vi "CB PWM Test.vi"(5 "HMP4040 Channel Settings":T2={"CH1 Voltage"=24.0, "CH1 Current"=1.0, "CH1 Output"=TRUE, "CH2 Voltage"=24.0, "CH2 Current"=1.0, "CH2 Output"=TRUE, "CH3 Voltage"=24.0, "CH3 Current"=1.0, "CH3 Output"=TRUE, "CH4 Voltage"=24.0, "CH4 Current"=1.0, "CH4 Output"=TRUE, "Master Output"=TRUE} {"CH4 Current" format="%.3f"; "CH4 Voltage" format="%.3f"; "CH3 Current" format="%.3f"; "CH3 Voltage" format="%.3f"; "CH2 Current" format="%.3f"; "CH2 Voltage" format="%.3f"; "CH1 Current" format="%.3f"; "CH1 Voltage" format="%.3f"}, 8 "error in (no error)":errorcluster, 9 "Board Selector":T1, 10 "Message IN":string=" ") -> (0 "error out":errorcluster, 1 "Result (bool)":bool, 2 "Message OUT":string, 3 "ControlBoard OUT":refnum<visa-resource-name>)   [LabVIEW 2022 SP3]
uses:
  HMP4000 Communication/HMP4040_ChannelControl.ctl
  Serial Board Com/Board Select.ctl
  <vilib>/DAQmx/read.llb/DAQmx Read (Analog 1D Wfm NChan NSamp).vi
  <vilib>/DAQmx/miscellaneous.llb/DAQmx Fill In Error Info.vi
panel:
  out "Analysis Leg":i32
  out "Waveforms":T3
  out "Active Leg":i32
  out "Result (color)":u32(colorbox)
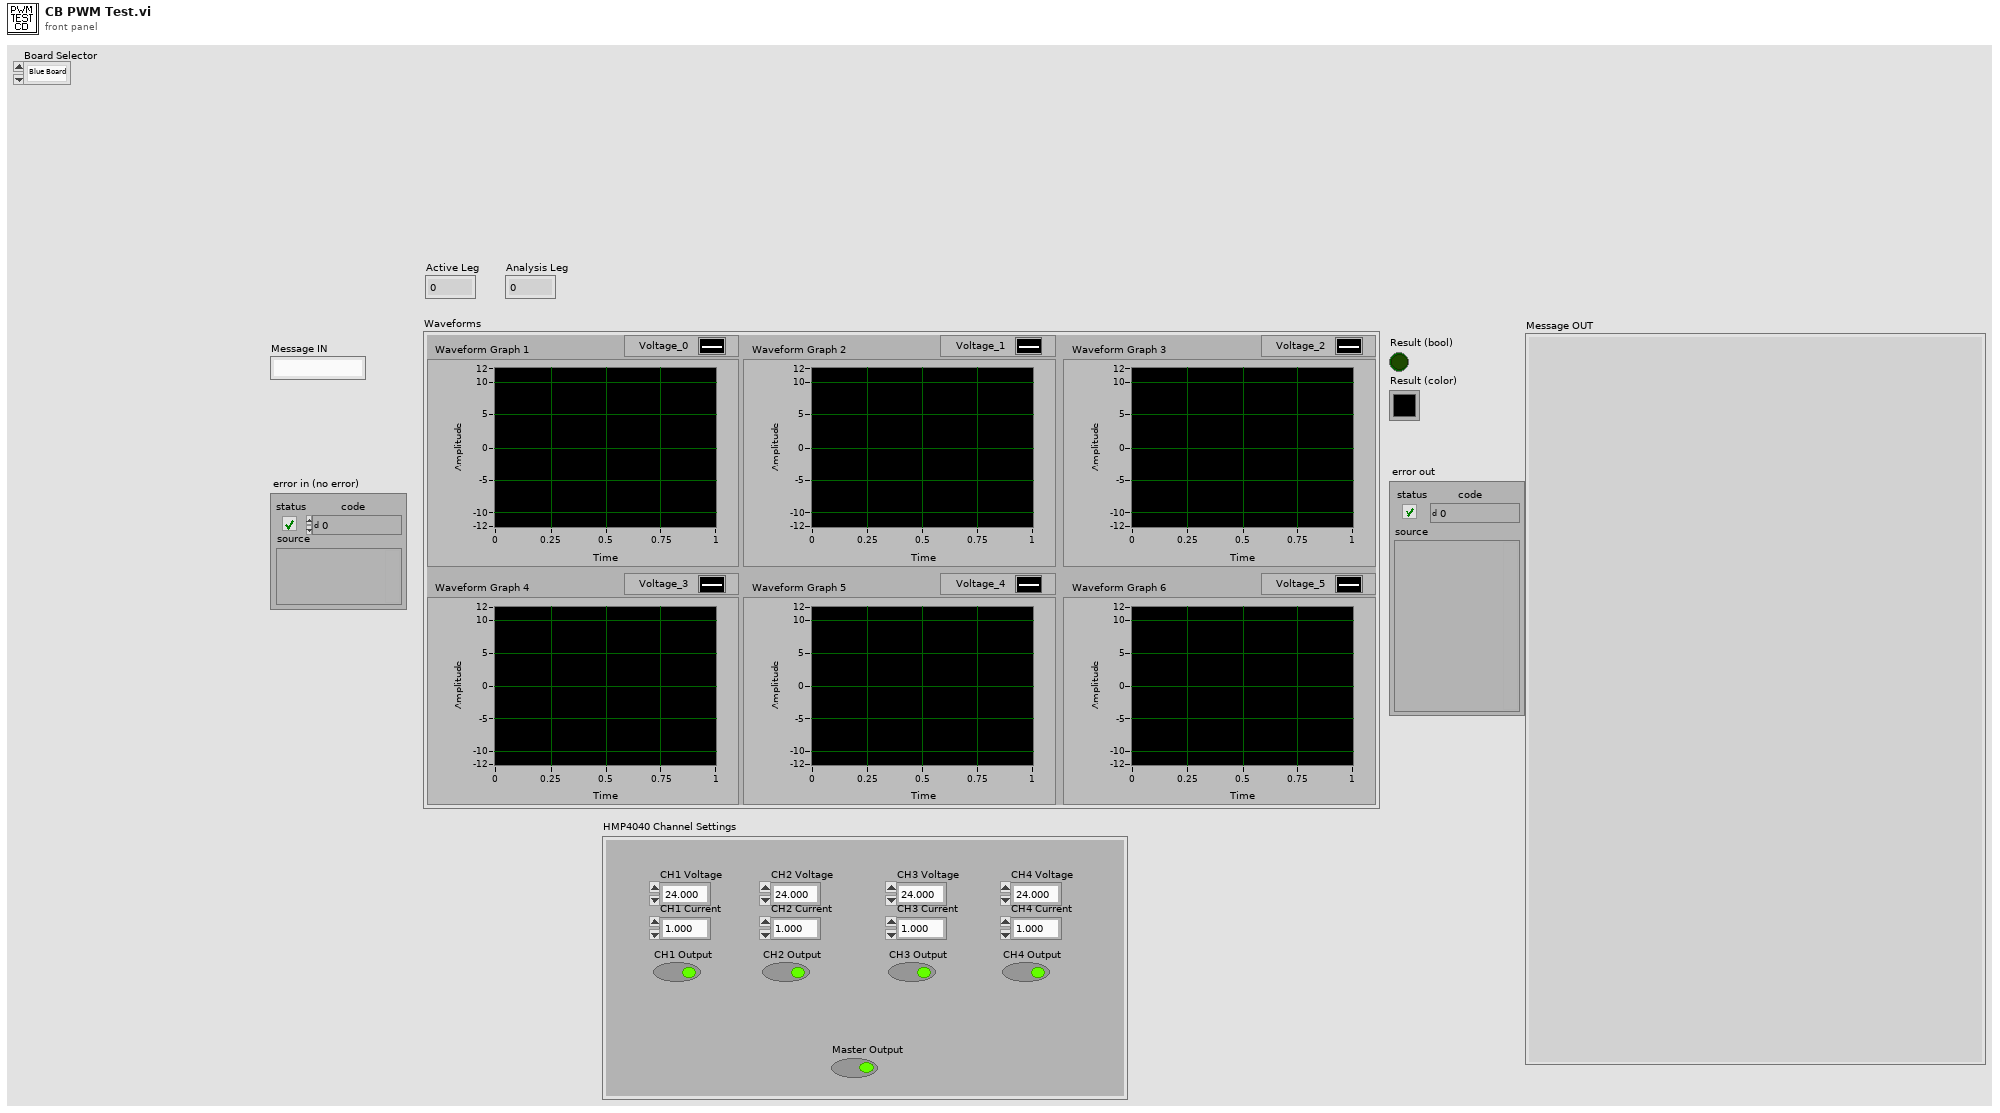
[diagram p1: front panel]
types:
  T1 = typedef "Board Select.ctl" = enum16{"Blue Board", "Green Board"}
  T2 = typedef "HMP4040_ChannelControl.ctl" = cluster{"CH1 Voltage":dbl, "CH1 Current":dbl, "CH1 Output":bool, "CH2 Voltage":dbl, "CH2 Current":dbl, "CH2 Output":bool, "CH3 Voltage":dbl, "CH3 Current":dbl, "CH3 Output":bool, "CH4 Voltage":dbl, "CH4 Current":dbl, "CH4 Output":bool, "Master Output":bool}
  T3 = cluster{"Waveform Graph 1":waveform(dbl), "Waveform Graph 2":waveform(dbl), "Waveform Graph 3":waveform(dbl), "Waveform Graph 4":waveform(dbl), "Waveform Graph 5":waveform(dbl), "Waveform Graph 6":waveform(dbl)}
  T4 = cluster{"data[0]":waveform(dbl), "data[1]":waveform(dbl), "data[2]":waveform(dbl), "data[3]":waveform(dbl), "data[4]":waveform(dbl), "data[5]":waveform(dbl)}
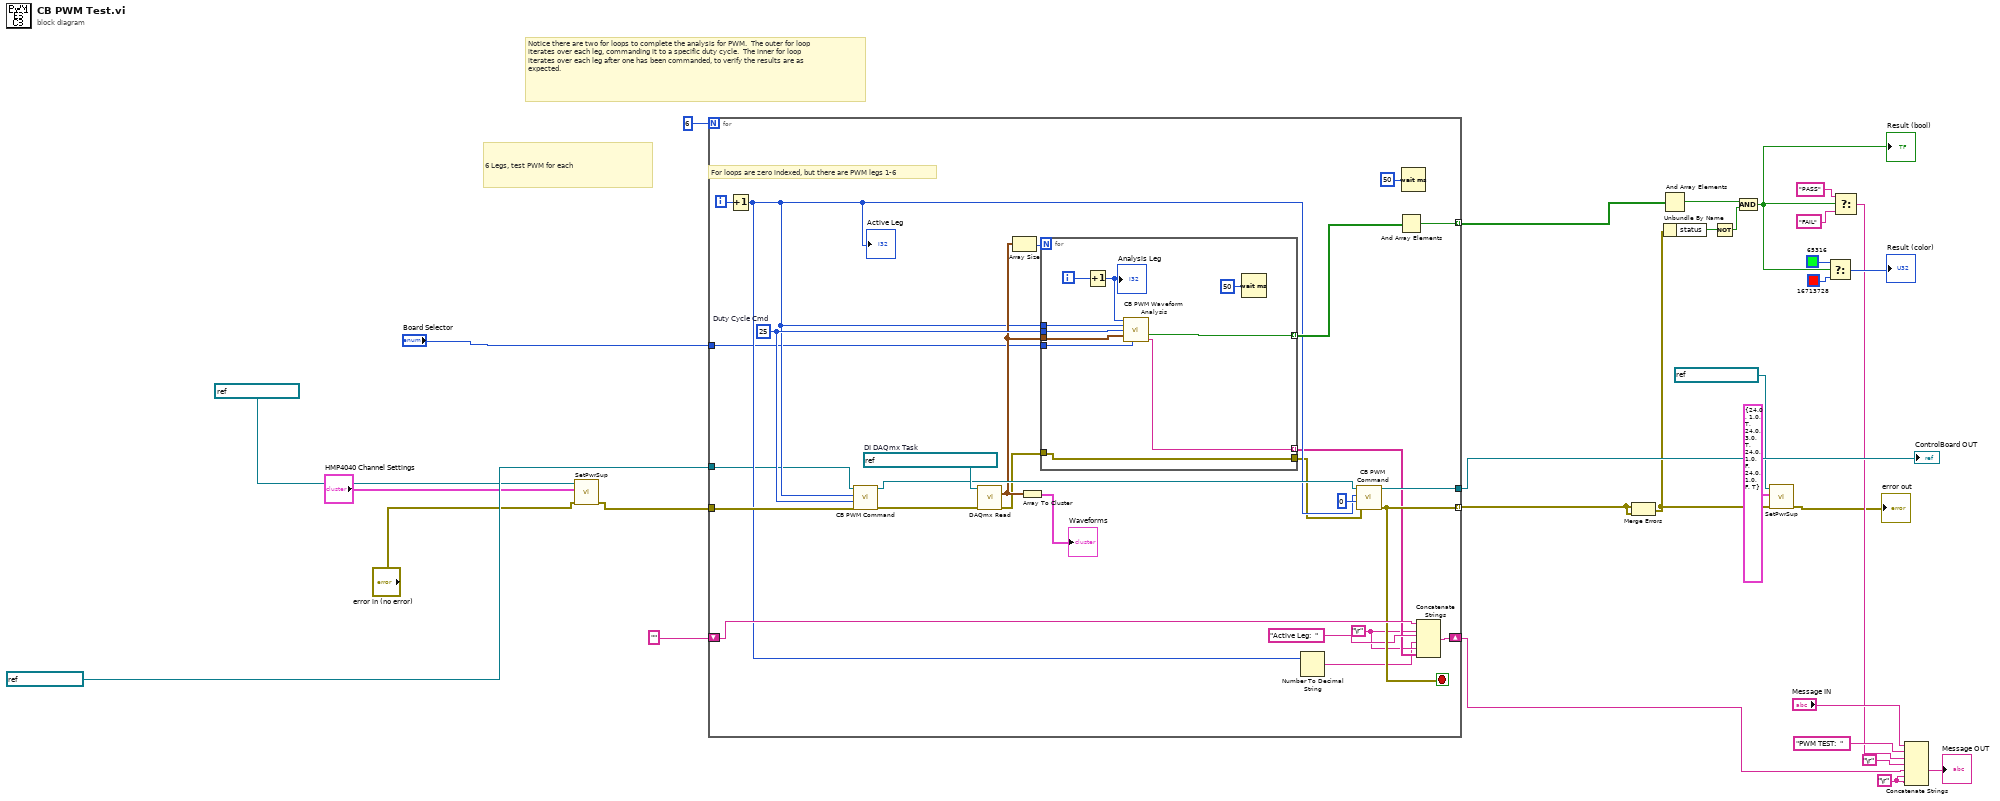
[diagram p0: block diagram]
diagram:
  w20 = "\r"
  # "Notice there are two for loops to complete the analysis for PWM.  The outer for loop iterates over each leg, commanding it to a specific duty cycle.  The inner for loop iterates over each leg after one has been commanded, to verify the results are as expected."
  # "6 Legs, test PWM for each"
  n1 = call "SetPwrSup.vi"("error in (no error)"="error in (no error)", "HMP4040 Channel Settings"="HMP4040 Channel Settings", "HMP4040 IN"=refnum<visa-resource-name> "HMP4040_FTS2" ("VISA resource name")) -> ("error out"=w8:errorcluster)  [unwired: 7 in, 1 out]
  n2 = for {
    N: 6 -> [_]
    tunnel: refnum<visa-resource-name> "ControlBoard" ("ControlBoard_IN") -> [w36]
    tunnel: [w57] -> w31 mode=indexing
    shift-right: [w54] -> w18
    shift-left: "" -> [w53]
    tunnel: w8 -> [w56]
    tunnel: [w48] -> w10 mode=indexing
    tunnel: [w43] -> w16
    tunnel: "Board Selector" -> [w35]
    i -> [w49]
    stop <- w48 stop-if-true
    w38 = "\r"
    w50 = 25  # Duty Cycle Cmd
    w55 = refnum<k21> "FTS2_PWMInput_Hydra_CB"  # DI DAQmx Task
    # "For loops are zero indexed, but there are PWM legs 1-6"
    n3 = Increment(x=w49) -> (x+1=w40:i32)
    "Active Leg" <- w40
    n4 = call "CB PWM Command.vi"("error in (no error)"=w56, "Duty Cycle"=w50, "Leg"=w40, "VISA Refnum in"=w36) -> ("error out"=w42:errorcluster, "VISA Refnum out"=w51:refnum<visa-resource-name>)  [unwired: 5 in, 1 out]
    n5 = call-poly <vilib>:"DAQmx Read.vi"("task/channels in"=w55, "error in"=w42) -> ("data"=w44:waveform(dbl)[], "error out"=w34:errorcluster)  [unwired: 11 in, 1 out]
    n6 = Array Size(array=w44) -> (size(s)=w45:i32)
    n7 = Array To Cluster(array=w44) -> (cluster=→"Waveforms":T4)
    n8 = for {
      N: w45 -> [_]
      tunnel: w50 -> [w67]
      tunnel: w44 -> [w66]
      tunnel: w40 -> [w65]
      tunnel: [w62] -> w46 mode=indexing
      tunnel: [w61] -> w39 mode=indexing
      tunnel: w35 -> [w59]
      tunnel: w34 -> [w60]
      tunnel: [w60] -> w33
      i -> [w64]
      n9 = Increment(x=w64) -> (x+1=w63:i32)
      "Analysis Leg" <- w63
      n10 = call "CB PWM Waveform Analysis.vi"("Analysis Leg"=w63, "Board Selector"=w59, "Active Leg"=w65, "Duty Cycle"=w67, "Waveform"=w66) -> ("Result (Boolean)"=w62:bool, "Message"=w61:string)  [unwired: 9 in]
      n11 = Wait (ms)(milliseconds to wait=u32 50) -> ()  [unwired: 1 out]
    }
    n12 = Number To Decimal String(number=w40) -> (decimal integer string=w37:string)  [unwired: 1 in]
    n13 = call "CB PWM Command.vi"("error in (no error)"=w33, "Duty Cycle"=0, "Leg"=w40, "VISA Refnum in"=w51) -> ("error out"=w48:errorcluster, "VISA Refnum out"=w43:refnum<visa-resource-name>)  [unwired: 5 in, 1 out]
    n14 = And Array Elements(Boolean array=w46) -> (logical AND=w57:bool)
    n15 = Wait (ms)(milliseconds to wait=u32 50) -> ()  [unwired: 1 out]
    n16 = Concatenate Strings(w53, w38, "Active Leg:  ", w37, w38, w39) -> (w54:string)
  }
  "ControlBoard OUT" <- w16
  n17 = Merge Errors(w10, w10) -> (w5:errorcluster)
  n18 = And Array Elements(Boolean array=w31) -> (logical AND=w21:bool)
  n19 = Unbundle By Name(w5) -> ("status"=w24:bool)
  n20 = Not(x=w24) -> (.not. x?=w23:bool)
  n21 = And(x=w21, y=w23) -> (x .and. y?=w22:bool)
  "Result (bool)" <- w22
  n22 = call "SetPwrSup.vi"("error in (no error)"=w5, "HMP4040 Channel Settings"=T2 {"CH1 Voltage"=24.0, "CH1 Current"=1.0, "CH1 Output"=TRUE, "CH2 Voltage"=24.0, "CH2 Current"=3.0, "CH2 Output"=TRUE, "CH3 Voltage"=24.0, "CH3 Current"=1.0, "CH3 Output"=FALSE, "CH4 Voltage"=24.0, "CH4 Current"=1.0, "CH4 Output"=FALSE, "Master Output"=TRUE}, "HMP4040 IN"=refnum<visa-resource-name> "HMP4040_FTS2" ("VISA resource name")) -> ("error out"=→"error out":errorcluster)  [unwired: 7 in, 1 out]
  n23 = Select(t=u32 65316 ("Result (color)"), s=w22, f=u32 16713728 ("Result (color)")) -> (s? t:f=→"Result (color)":u32)
  n24 = Select(t="PASS", s=w22, f="FAIL") -> (s? t:f=w12:string)
  n25 = Concatenate Strings("Message IN", "PWM TEST:  ", w12, "\r", w18, w20, w20) -> (→"Message OUT":string)
